vi "RT Main.vi"() -> ()   [LabVIEW 2021]
panel:
  out "# elements in queue":i32
  out "Elements in queue":i32[](array[numeric])
  out "Dequeue elements":i32
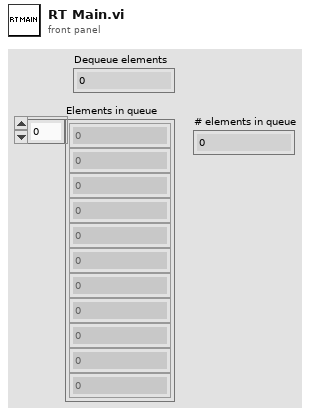
[diagram p1: front panel]
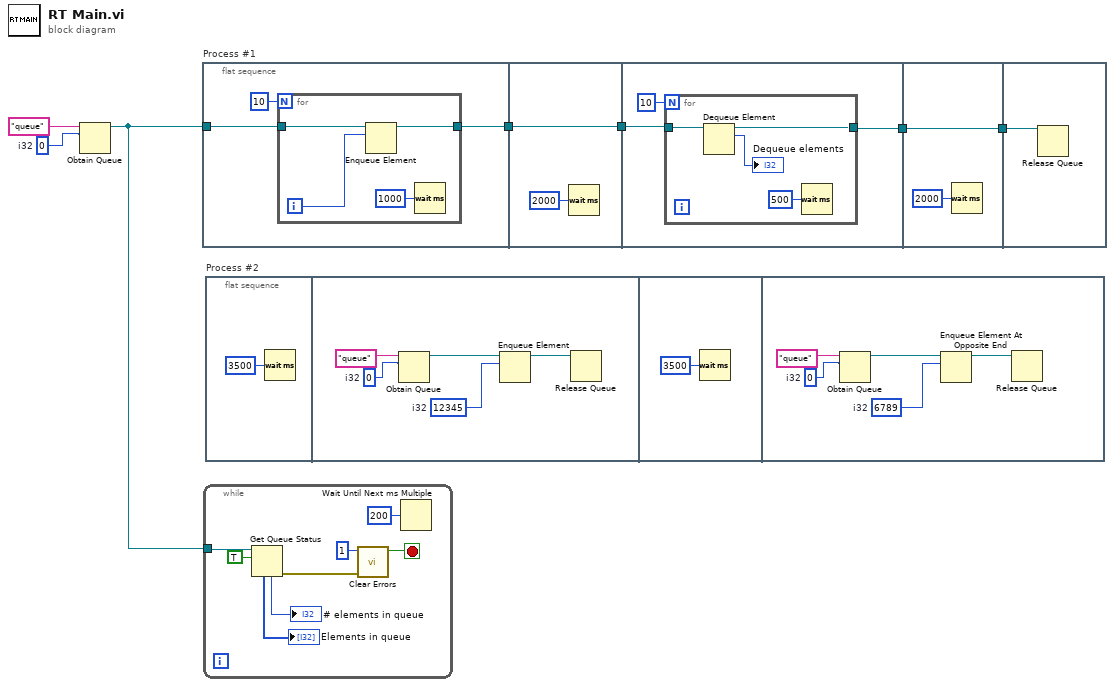
[diagram p0: block diagram]
diagram:
  w7 = 0  # i32
  n1 = Obtain Queue(name (unnamed)="queue", element data type=w7) -> (queue out=w2:refnum<queue>)  [unwired: 3 in, 2 out]
  n2 = flat-sequence "Process #1" {
    tunnel: w2 -> [w9]
    tunnel: [w8] -> w6
    tunnel: w6 -> [w15]
    tunnel: [w15] -> w5
    tunnel: w5 -> [w19]
    tunnel: [w18] -> w3
    tunnel: [w24] -> w4
    tunnel: w3 -> [w24]
    tunnel: w4 -> [w26]
    frame #0 {
      n3 = for {
        N: 10 -> [_]
        tunnel: w9 -> [w14]
        tunnel: [w11] -> w8
        i -> [w13]
        n4 = Enqueue Element(queue=w14, element=w13) -> (queue out=w11:refnum<queue>)  [unwired: 2 in, 2 out]
        n5 = Wait (ms)(milliseconds to wait=u32 1000) -> ()  [unwired: 1 out]
      }
    }
    frame #1 {
      n6 = Wait (ms)(milliseconds to wait=u32 2000) -> ()  [unwired: 1 out]
    }
    frame #2 {
      n7 = for {
        N: 10 -> [_]
        tunnel: w19 -> [w23]
        tunnel: [w21] -> w18
        n8 = Dequeue Element(queue=w23) -> (queue out=w21:refnum<queue>, element=→"Dequeue elements":i32)  [unwired: 2 in, 2 out]
        n9 = Wait (ms)(milliseconds to wait=u32 500) -> ()  [unwired: 1 out]
      }
    }
    frame #3 {
      n10 = Wait (ms)(milliseconds to wait=u32 2000) -> ()  [unwired: 1 out]
    }
    frame #4 {
      n11 = Release Queue(queue=w26) -> ()  [unwired: 2 in, 3 out]
    }
  }
  n12 = while {
    tunnel: w2 -> [w34]
    stop <- w30 stop-if-true
    n13 = Get Queue Status(queue=w34, return elements? (F)=TRUE) -> (error out=w32:errorcluster, # elements in queue=→"# elements in queue":i32, elements=→"Elements in queue":i32[])  [unwired: 1 in, 5 out]
    n14 = call <vilib>:"Clear Errors.vi"("error in (no error)"=w32, "specific error code to clear (0: all)"=1) -> ("specific error cleared?"=w30:bool)  [unwired: 4 in, 1 out]
    n15 = Wait Until Next ms Multiple(millisecond multiple=u32 200) -> ()  [unwired: 1 out]
  }
  n16 = flat-sequence "Process #2" {
    frame #0 {
      n17 = Wait (ms)(milliseconds to wait=u32 3500) -> ()  [unwired: 1 out]
    }
    frame #1 {
      w37 = 12345  # i32
      w39 = 0  # i32
      n18 = Obtain Queue(name (unnamed)="queue", element data type=w39) -> (queue out=w38:refnum<queue>)  [unwired: 3 in, 2 out]
      n19 = Enqueue Element(queue=w38, element=w37) -> (queue out=w36:refnum<queue>)  [unwired: 2 in, 2 out]
      n20 = Release Queue(queue=w36) -> ()  [unwired: 2 in, 3 out]
    }
    frame #2 {
      n21 = Wait (ms)(milliseconds to wait=u32 3500) -> ()  [unwired: 1 out]
    }
    frame #3 {
      w45 = 6789  # i32
      w43 = 0  # i32
      n22 = Obtain Queue(name (unnamed)="queue", element data type=w43) -> (queue out=w44:refnum<queue>)  [unwired: 3 in, 2 out]
      n23 = Enqueue Element At Opposite End(queue=w44, element=w45) -> (queue out=w46:refnum<queue>)  [unwired: 2 in, 2 out]
      n24 = Release Queue(queue=w46) -> ()  [unwired: 2 in, 3 out]
    }
  }
